vi "Design FIR filter.vi"(4 "optional FIR filter specifications":T2={"PB Gain"=3.0, "SB Gain"=60.0, "Scale"=TRUE, "Window"=enum."Flat Top"} {"SB Gain" format="%0.2f"; "PB Gain" format="%0.2f"}, 6 "FIR filter specifications":T3={"Topology"=enum."Off", "Type"=enum."Bandstop", "#Taps"=1500, "Lower PB"=1500.0, "Upper PB"=1500.0, "Lower SB"=0.0, "Upper SB"=0.0} {"Lower SB" format="%0.2p"; "Upper SB" format="%0.2p"; "Lower PB" format="%0.2p"; "Upper PB" format="%0.2p"}, 7 "redesign filter":bool, 8 "error in":errorcluster, 11 "dt":dbl format="%0.2f") -> (0 "error out":errorcluster, 1 "forward coefficients":dbl[](array[numeric]) format="%0.2f", 3 "filter information":T1 {"phase H(w)"."df" format="%0.2f"; "phase H(w)"."f0" format="%0.2f"; "phase H(w)"."Phase H(w)" format="%0.2f"; "magnitude H(w)"."df" format="%0.2f"; "magnitude H(w)"."f0" format="%0.2f"; "magnitude H(w)"."Mag H(w)" format="%0.2f"}, 5 "reset filter state":bool)   [LabVIEW 2020, in "NI_MAPro.lvlib"]
uses:
  NI_MAPro.lvlib
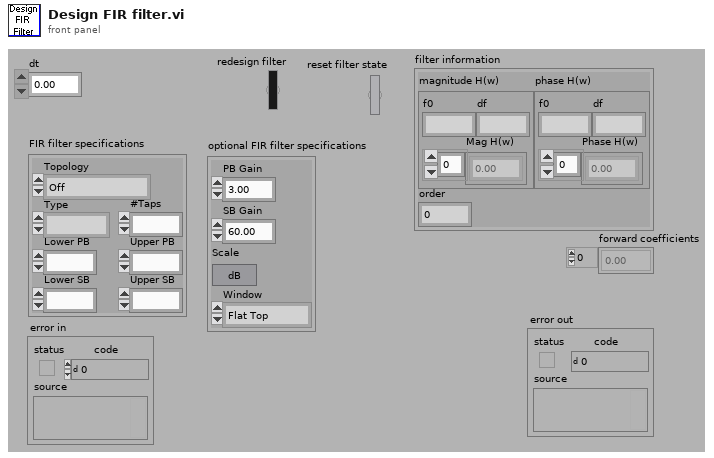
[diagram p1: front panel]
types:
  T1 = cluster{"magnitude H(w)":cluster{"f0":dbl, "df":dbl, "Mag H(w)":dbl[]}, "phase H(w)":cluster{"f0":dbl, "df":dbl, "Phase H(w)":dbl[]}, "order":i32}
  T2 = cluster{"PB Gain":dbl, "SB Gain":dbl, "Scale":bool, "Window":enum16{"None", "Hanning", "Hamming", "Triangular", "Blackman", "Exact Blackman", "Blackman-Harris", "Kaiser-Bessel", "Flat Top"}}
  T3 = cluster{"Topology":enum16{"Off", "FIR by Specification", "Equi-ripple FIR", "Windowed FIR"}, "Type":enum16{"Lowpass", "Highpass", "Bandpass", "Bandstop"}, "#Taps":i32, "Lower PB":dbl, "Upper PB":dbl, "Lower SB":dbl, "Upper SB":dbl}
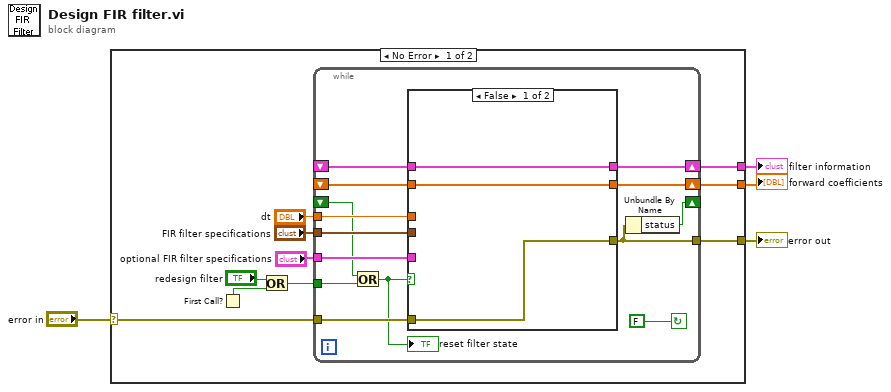
[diagram p0: block diagram]
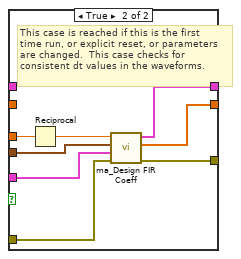
[diagram p2: hidden frame]
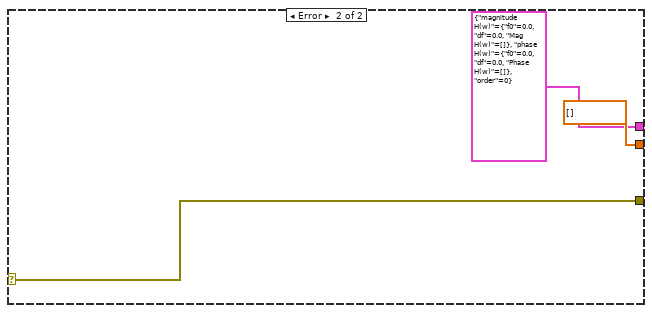
[diagram p3: hidden frame]
diagram:
  n1 = case shown="No Error" "error in" {
    selector: "error in" -> [w13 w42]
    tunnel: [w14 w42] -> w4
    tunnel: [w12 dbl[] [] ("Forward Coefficients")] -> w2
    tunnel: [w11 T1 {"magnitude H(w)"={"f0"=0.0, "df"=0.0, "Mag H(w)"=[]}, "phase H(w)"={"f0"=0.0, "df"=0.0, "Phase H(w)"=[]}, "order"=0} ("Filter Information")] -> w1
    frame No Error {
      n2 = First Call?() -> (First Call?: T/F=w9:bool)
      n3 = Or(x="redesign filter", y=w9) -> (x .or. y?=w8:bool)
      n4 = while {
        tunnel: "dt" -> [w20]
        tunnel: "FIR filter specifications" -> [w22]
        tunnel: "optional FIR filter specifications" -> [w23]
        tunnel: w13 -> [w21]
        tunnel: [w19] -> w14
        shift-left: _ -> [w26]
        shift-right: [w27] -> w12
        shift-left: _ -> [w24]
        shift-right: [w25] -> w11
        tunnel: w8 -> [w17]
        shift-right: [w18] -> _
        shift-left: _ -> [w16]
        stop <- FALSE continue-if-true
        n5 = Or(x=w16, y=w17) -> (x .or. y?=w15:bool)
        "reset filter state" <- w15
        n6 = case shown="False" w15 {
          tunnel: w24 -> [w31 _]
          tunnel: [w30 w32] -> w27
          tunnel: w26 -> [w30 _]
          tunnel: [w31 w33] -> w25
          tunnel: [w29 w38] -> w19
          tunnel: w20 -> [_ w39]
          tunnel: w22 -> [_ w36]
          tunnel: w23 -> [_ w35]
          tunnel: w21 -> [w29 w37]
          frame False {
            # "No change in parameters, no reset, and not the first time run."
          }
          frame True {
            # "This case is reached if this is the first\ntime run, or explicit reset, or parameters \nare changed.  This case checks for\nconsistent dt values in the waveforms."
            n7 = Reciprocal(x=w39) -> (1/x=w34:dbl)
            n8 = call "ma_Design FIR Coeff.vi"("error in"=w37, "Optional FIR Filter Specifications"=w35, "FIR Filter Specifications"=w36, "Sampling Frequency"=w34) -> ("error out"=w38:errorcluster, "Forward Coefficients"=w32:dbl[], "Filter Information"=w33:T1)  [unwired: 5 in]
          }
        }
        n9 = Unbundle By Name(w19) -> ("status"=w18:bool)
      }
    }
    frame Error {
    }
  }
  "error out" <- w4
  "forward coefficients" <- w2
  "filter information" <- w1
